vi "gyro-sweeper-V3.vi"() -> ()   [LabVIEW 2018]
uses:
  filename-pattern.ctl
  show-win- control.ctl
  cursor winow.ctl
  cursor window action.ctl
  server talkto message type.ctl
  server talkback message type.ctl
  server talk-to-back pair.ctl
  pll internal user event action.ctl
  publisher action.ctl
  file -- read-write control.ctl
  KM_file -- read-write control.ctl
  filename-action.ctl
  <vilib>/Analysis/baseanly.llb/A x B.vi
  <vilib>/Analysis/baseanly.llb/Complex A x B.vi
  Q -- check range -- i -- real.vi
  line -- complex.vi
  Q -- check range -- i -- integer.vi
  Q - not nan -- real.vi
  Q - not nan -- integer.vi
  <vilib>/Analysis/Matrix/Numeric/Conversions/Array To Matrix.vi
  <vilib>/Analysis/Matrix/Numeric/Conversions/Array To Matrix - RA2.vi
  <vilib>/Analysis/baseanly.llb/Inverse Matrix.vi
  <vilib>/Analysis/baseanly.llb/Real Inverse Matrix.vi
panel:
  in  "(*) sourcer":bool
  in  "exit!":bool
  in  "(*) fitter":bool
  in  "(*) sweeper":bool=TRUE
  in  "sweeper panel":T1(tab)
  in  "sweep is ON":bool
  in  "win":T2={"cen (Hz)"=32754.180483243686, "win (Hz)"=308.86311527720136, "left (Hz)"=32599.748925605087, "right (Hz)"=32908.61204088229}
  out "Plot: circle sweep window":cluster{"Freq out (Hz)":dbl[], dbl[]}[](graph)
  in  "sweep! :r":bool
  in  "subtract bgnd!":bool
  in  "fit!":bool=TRUE
  in  "cursor window":T3={"left"=32599.748925605087, "right "=32908.61204088229, "center"=32754.180483243686, "window"=308.86311527720136, "cursors"=[0, 1, 2], "relative"=0, "absolute"=0, "fixed vertical offset"=0.0, "vertical offset"=0.0, "skew"=0.0, "default window frac"=0.1, "kind"=enum."symmetric", "skew.left"=0.5, "skew.right"=0.5, "Plot ref"=refnum, "wing order"=enum."forw"}
  out "async sweeper":refnum<vi>
  out "async fitter":refnum<vi>
  out "async sourcer":refnum<vi>
  in  "view/hide sweeper 2":bool=TRUE
  in  "view/hide fitter 2":bool
  in  "view/hide sourcer 2":bool
  in  "save data":enum32{"save/read"}(tab)
  in  "freqsweep name template":T4={"prefix"="RuCl3-rod", "group"="f"}
  in  "Save folder":path=path "/Users/Shared/Data"
  in  "freq sweep file name":string="f020_RuCl3-rod_042518.dat"
  in  "read from disk :l":bool
  in  "read file":path=path "/Users/arkady/Desktop/local_data/TaAs-quirk-Jan2018-losalamos/9w/f006_rucl3_012518.dat"
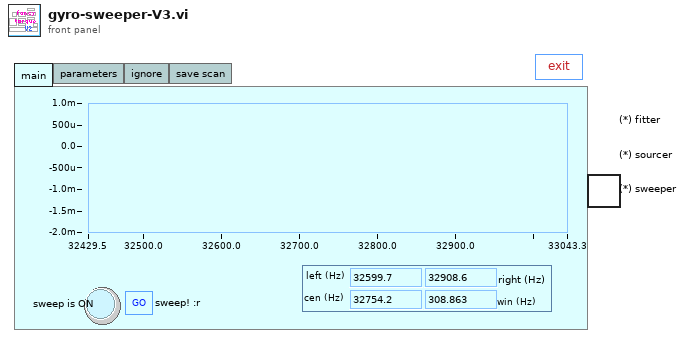
[diagram p1: front panel]
types:
  T1 = enum32{"main", "parameters", "ignore", "save scan"}
  T2 = typedef "show-win- control.ctl" = cluster{"cen (Hz)":dbl, "win (Hz)":dbl, "left (Hz)":dbl, "right (Hz)":dbl}
  T3 = typedef "cursor winow.ctl" = cluster{"left":dbl, "right ":dbl, "center":dbl, "window":dbl, "cursors":i32[], "relative":i32, "absolute":i32, "fixed vertical offset":dbl, "vertical offset":dbl, "skew":dbl, "default window frac":dbl, "kind":enum16{"symmetric", "skewed", "fancy"}, "skew.left":dbl, "skew.right":dbl, "Plot ref":refnum<vi>, "wing order":enum16{"forw", "back"}}
  T4 = typedef "filename-pattern.ctl" = cluster{"prefix":string, "group":string}
  T5 = typedef "server talk-to-back pair.ctl" = cluster{"talkback event":refnum<user-event>, "talkto event":refnum<user-event>}
  T6 = typedef "server talkback message type.ctl" = cluster{"message":enum16{"new"}}
  T7 = typedef "server talkto message type.ctl" = cluster{"message":enum16{"stop", "start", "update pars", "update request", "new", "launch", "exit", "get", "reset", "pause", "unpause"}}
  T8 = typedef "pll internal user event action.ctl" = enum16{"gear pll async", "start pll async", "stop pll async", "toggle pll async", "gear sweeper", "start sweeper", "stop sweeper", "toggle sweeper", "accept frequency", "reset lorentzian", "accept lorentzian", "update cursors", "pause pll", "unpause pll", "void"}
  T9 = typedef "cursor window action.ctl" = enum16{"balance", "h. offset change", "cursor moves", "change center", "change window", "init", "check", "reset", "set y to middle", "idle", "-write all Y", "-write left.X", "-write center.X", "-write right.X", "-write all X", "-change center", "-change window", "-change skew", "-read cursor 2", "-read cursor 1", "-read cursor 0", "-read all cursors", "-reset", "-read plot scale", "-set y to middle", "-Q: center.Y is visible", "-Q: window is visible", "-parse center.Y", "-right left from center", "-left move", "-right move", "-set center.Y", "-empty", "-set cursors to default", "-check", "-write center.Y", "-copy cursor 1", "-copy cursor 0", "-copy cursor 2", "move right", "move left", "shrink", "broaden", "skew up", "skew down", "-write plot scale", "zoom X", "change cen&win", "zoom to all data", "color--red", "color--green", "color--yellow", "read", "zoom out", "zoom in", "slide right", "slide left", "set range aspect ratio to 1"}
  T10 = typedef "eventvkey.ctl" = enum16{"ASCII", "Enter", "Return", "Shift", "Ctrl", "Alt", "Cmd", "Opt", "Caps", "NumLock", "Clear", "Break", "Up", "Down", "Left", "Right", "Insert", "Delete", "Home", "End", "PageUp", "PageDown", "Escape", "Help", "Pause", "ScrollLock", "F1", "F2", "F3", "F4", "F5", "F6", "F7", "F8", "F9", "F10", "F11", "F12", "F13", "F14", "F15", "F16", "F17", "F18", "F19", "F20", "F21", "F22", "F23", "F24", "Play", "VolumeUp", "VolumeDown", "Mute", "Two Byte Char"}
  T11 = typedef "publisher action.ctl" = enum16{"set", "get", "init", "check"}
  T12 = typedef "file -- read-write control.ctl" = enum16{"read", "write all", "append one line"}
  T13 = typedef "filename-action.ctl" = enum16{"rewrite", "parse", "force pattern", "uniquenum"}
  T14 = typedef "KM_file -- read-write control.ctl" = enum16{"read", "write all", "append one line"}
  T15 = enum32{"Invalid", "Standard", "Closed", "Hidden", "Minimized", "Maximized"}
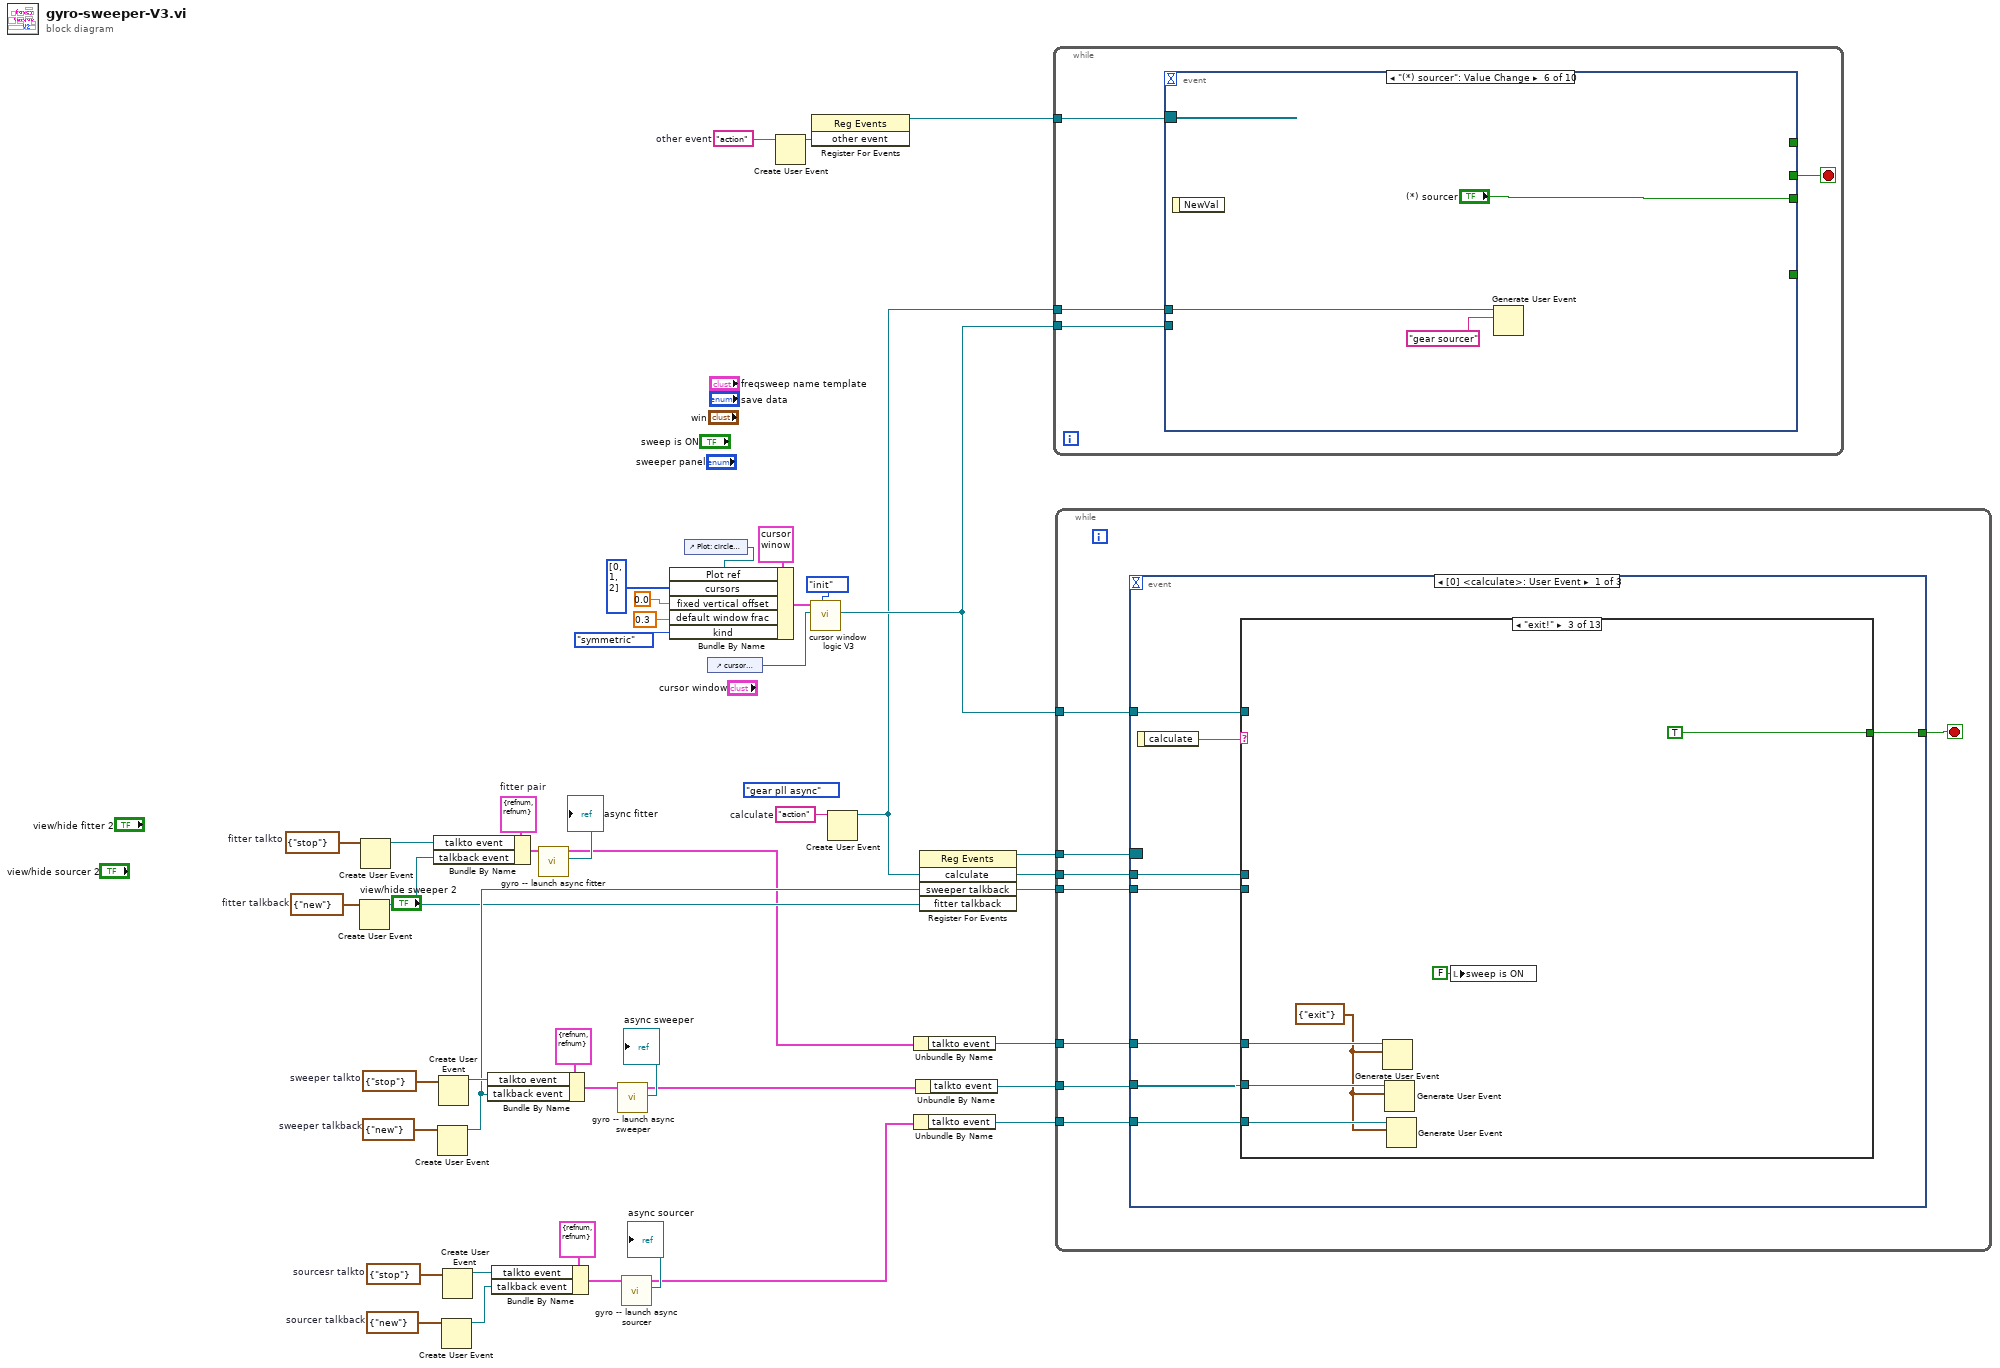
[diagram p0: block diagram]
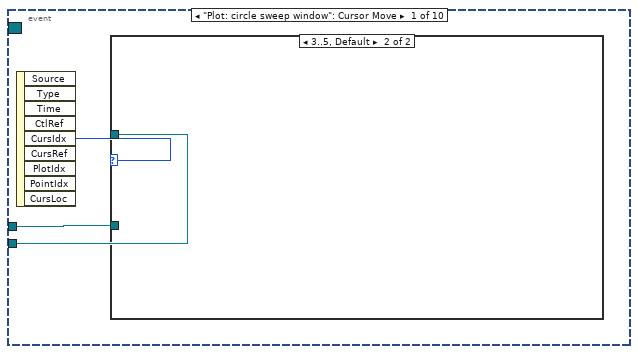
[diagram p2: hidden frame]
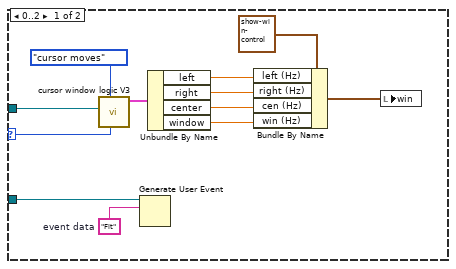
[diagram p3: hidden frame]
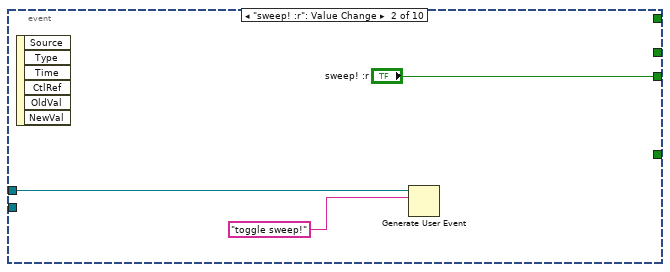
[diagram p4: hidden frame]
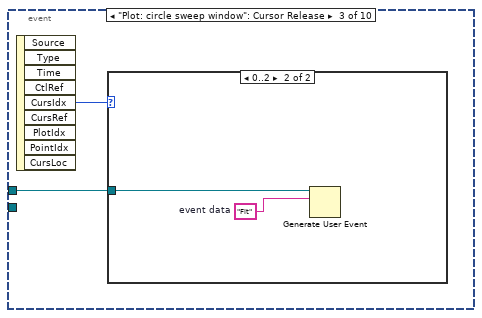
[diagram p5: hidden frame]
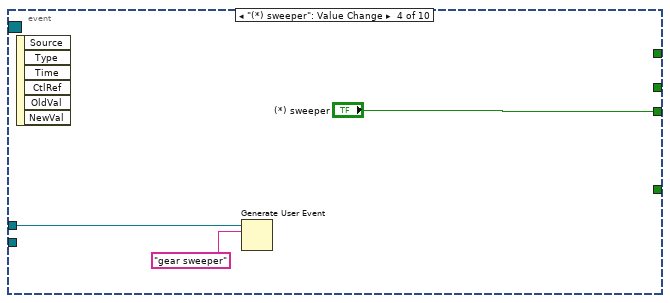
[diagram p7: hidden frame]
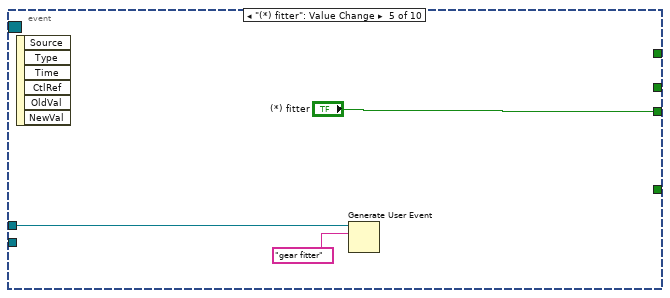
[diagram p8: hidden frame]
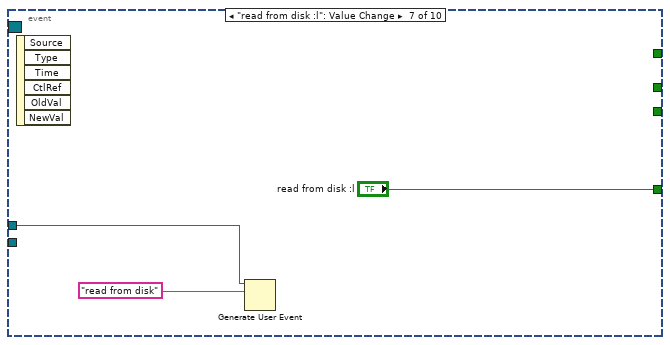
[diagram p9: hidden frame]
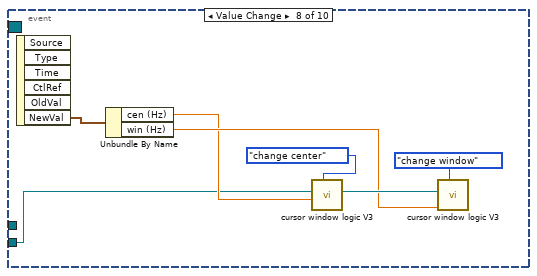
[diagram p10: hidden frame]
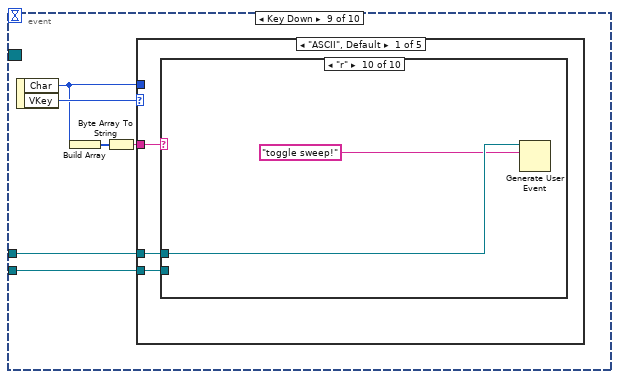
[diagram p11: hidden frame]
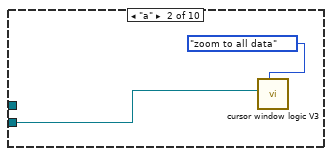
[diagram p13: hidden frame]
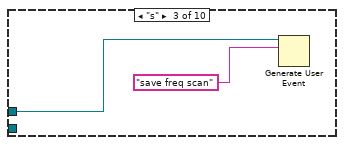
[diagram p14: hidden frame]
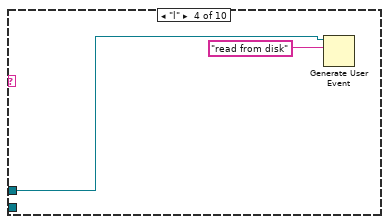
[diagram p15: hidden frame]
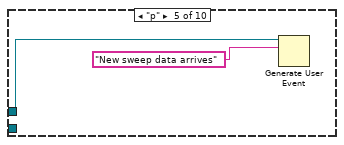
[diagram p16: hidden frame]
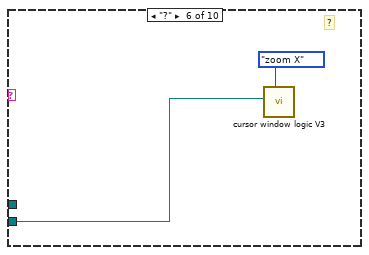
[diagram p17: hidden frame]
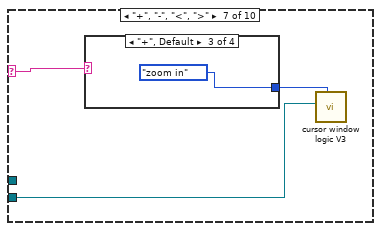
[diagram p18: hidden frame]
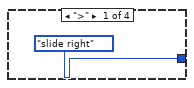
[diagram p19: hidden frame]
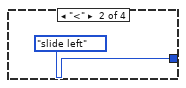
[diagram p20: hidden frame]
diagram:
  w5 = T6 {"message"=enum."new"}  # sourcer talkback
  w6 = T7 {"message"=enum."stop"}  # sourcesr talkto
  w17 = T6 {"message"=enum."new"}  # sweeper talkback
  w18 = T7 {"message"=enum."stop"}  # sweeper talkto
  w26 = T5 {"talkback event"=refnum, "talkto event"=refnum}  # fitter pair
  w15 = T6 {"message"=enum."new"}  # fitter talkback
  w16 = T7 {"message"=enum."stop"}  # fitter talkto
  (unwired) pll_internal_user_event_action."gear pll async" ("pll event action")
  w40 = "action"  # other event
  w42 = "action"  # calculate
  n1 = Create User Event(user event datatype=w15) -> (user event=w12:refnum<user-event>)  [unwired: 1 in, 1 out]
  n2 = Create User Event(user event datatype=w16) -> (user event=w25:refnum<user-event>)  [unwired: 1 in, 1 out]
  n3 = Bundle By Name(cluster=w26, "talkto event"=w25, "talkback event"=w12) -> (w19:T5)
  n4 = Create User Event(user event datatype=w17) -> (user event=w13:refnum<user-event>)  [unwired: 1 in, 1 out]
  n5 = Create User Event(user event datatype=w18) -> (user event=w23:refnum<user-event>)  [unwired: 1 in, 1 out]
  n6 = Create User Event(user event datatype=w5) -> (user event=w3:refnum<user-event>)  [unwired: 1 in, 1 out]
  n7 = Create User Event(user event datatype=w6) -> (user event=w8:refnum<user-event>)  [unwired: 1 in, 1 out]
  n8 = Bundle By Name(cluster=T5 {"talkback event"=refnum, "talkto event"=refnum} ("sweeper pair"), "talkto event"=w23, "talkback event"=w13) -> (w14:T5)
  n9 = Bundle By Name(cluster=T5 {"talkback event"=refnum, "talkto event"=refnum} ("sweeper pair"), "talkto event"=w8, "talkback event"=w3) -> (w4:T5)
  n10 = call "gyro -- launch async fitter.vi"("fitter pair"=w19) -> ("reference out"=→"async fitter":refnum<vi>, "fitter pair OUT"=w10:T5)  [unwired: 9 in]
  n11 = call "gyro -- launch async sweeper.vi"("sweeper event pair"=w14) -> ("reference out"=→"async sweeper":refnum<vi>, "sweeper event pair OUT"=w11:T5)  [unwired: 9 in]
  n12 = call "gyro -- launch async sourcer.vi"("sourcer pair"=w4) -> ("reference out"=→"async sourcer":refnum<vi>, "fitter pair OUT"=w2:T5)  [unwired: 9 in]
  n13 = control-ref of="Plot: circle sweep window"() -> (w29:refnum<vi>)
  n14 = Bundle By Name(cluster=T3 {"left"=0.0, "right "=0.0, "center"=0.0, "window"=0.0, "cursors"=[], "relative"=0, "absolute"=0, "fixed vertical offset"=0.0, "vertical offset"=0.0, "skew"=0.0, "default window frac"=0.0, "kind"=enum."symmetric", "skew.left"=0.0, "skew.right"=0.0, "Plot ref"=refnum, "wing order"=enum."forw"} ("cursor bracket: All, data window"), "Plot ref"=w29, "cursors"=i32[] [0, 1, 2], "fixed vertical offset"=0.0, "default window frac"=0.3 ("fixed vertical offset"), "kind"=enum16{"symmetric", "skewed", "fancy"}."symmetric") -> (w34:T3)
  n15 = control-ref of="cursor window"() -> (w27:refnum<vi>)
  n16 = Create User Event(user event datatype=w40) -> (user event=w39:refnum<user-event>)  [unwired: 1 in, 1 out]
  n17 = call "cursor window logic V3.vi"("cursor window action"=cursor_window_action."init", "cursor window in"=w27, "cursor window init"=w34) -> ("cursor window out"=w32:refnum<vi>)  [unwired: 7 in, 1 out]
  n18 = register-events(w39) -> (reference out=w41:refnum<event-registration>)  [unwired: 2 in, 1 out]
  n19 = Create User Event(user event datatype=w42) -> (user event=w30:refnum<user-event>)  [unwired: 1 in, 1 out]
  n20 = Unbundle By Name(w10) -> ("talkto event"=w21:refnum<user-event>)
  n21 = Unbundle By Name(w2) -> ("talkto event"=w1:refnum<user-event>)
  n22 = Unbundle By Name(w11) -> ("talkto event"=w22:refnum<user-event>)
  n23 = register-events(w30, w13, w12) -> (reference out=w43:refnum<event-registration>)  [unwired: 2 in, 1 out]
  n24 = while {
    tunnel: w41 -> [w47]
    tunnel: w30 -> [w46]
    tunnel: w32 -> [w45]
    stop <- w44 stop-if-true
    n25 = event shown="[5] \"(*) sourcer\": Value Change" {
      selector: w47 -> [_ _ _ _ _ _ _ _ _ _]
      dyn-events: _ -> [_ _ _ _ _ _ _ _ _ _]
      timeout: _ -> [_ _ _ _ _ _ _ _ _ _]
      tunnel: w46 -> [w48 w64 w67 w71 w73 w76 w81 _ w93 w138]
      tunnel: w45 -> [w50 _ _ _ _ _ _ w82 w89 _]
      tunnel: [_ "sweep! :r" _ "(*) sweeper" "(*) fitter" "(*) sourcer" _ _ _ _] -> _
      tunnel: [_ _ _ _ _ _ "read from disk :l" _ _ _] -> _
      tunnel: [_ _ _ _ _ _ _ _ _ "exit!"] -> _
      tunnel: [_ _ _ _ _ _ _ _ _ TRUE] -> w44
      event "Plot: circle sweep window": Cursor Move {
        n26 = event-data() -> ("CursIdx"=w49:i32)  [unwired: 1 in, 8 out]
        n27 = case shown="3..5, Default" w49 {
          selector: w49 -> [w60 _]
          tunnel: w50 -> [w62 _]
          tunnel: w48 -> [w58 _]
          frame 0..2 {
            w57 = "Fit"  # event data
            n28 = call "cursor window logic V3.vi"("CursIdx"=w60, "cursor window action"=cursor_window_action."cursor moves", "cursor window in"=w62) -> ("cursor window out"=w59:T3)  [unwired: 7 in, 1 out]
            n29 = Generate User Event(user event=w58, event data cluster=w57) -> ()  [unwired: 2 in, 2 out]
            n30 = Unbundle By Name(w59) -> ("left"=w54:dbl, "right"=w53:dbl, "center"=w52:dbl, "window"=w51:dbl)
            n31 = Bundle By Name(cluster=T2 {"cen (Hz)"=-0.35260838541595674, "win (Hz)"=17.234446484426172, "left (Hz)"=-8.969831627629043, "right (Hz)"=8.26461485679713} ("win"), "left (Hz)"=w54, "right (Hz)"=w53, "cen (Hz)"=w52, "win (Hz)"=w51) -> (w55:T2)
            n32 = local write "win"(w55) -> ()
          }
          frame 3..5, Default {
          }
        }
      }
      event "sweep! :r": Value Change {
        n33 = event-data() -> ()  [unwired: 1 in, 6 out]
        n34 = Generate User Event(user event=w64, event data cluster="toggle sweep!" ("event data")) -> ()  [unwired: 2 in, 2 out]
      }
      event "Plot: circle sweep window": Cursor Release {
        n35 = event-data() -> ("CursIdx"=w66:i32)  [unwired: 1 in, 8 out]
        n36 = case shown="0..2" w66 {
          tunnel: w67 -> [_ w68]
          frame 3, Default {
          }
          frame 0..2 {
            w69 = "Fit"  # event data
            n37 = Generate User Event(user event=w68, event data cluster=w69) -> ()  [unwired: 2 in, 2 out]
          }
        }
      }
      event "(*) sweeper": Value Change {
        n38 = event-data() -> ()  [unwired: 1 in, 6 out]
        n39 = Generate User Event(user event=w71, event data cluster="gear sweeper" ("event data")) -> ()  [unwired: 2 in, 2 out]
      }
      event "(*) fitter": Value Change {
        n40 = event-data() -> ()  [unwired: 1 in, 6 out]
        n41 = Generate User Event(user event=w73, event data cluster="gear fitter" ("event data")) -> ()  [unwired: 2 in, 2 out]
      }
      event "(*) sourcer": Value Change {
        n42 = event-data() -> ()  [unwired: 1 in, 1 out]
        n43 = Generate User Event(user event=w76, event data cluster="gear sourcer" ("event data")) -> ()  [unwired: 2 in, 2 out]
      }
      event "read from disk :l": Value Change {
        n44 = event-data() -> ()  [unwired: 1 in, 6 out]
        n45 = Generate User Event(user event=w81, event data cluster="read from disk" ("event data")) -> ()  [unwired: 2 in, 2 out]
      }
      event Value Change {
        n46 = event-data() -> ("NewVal"=w85:T2)  [unwired: 1 in, 5 out]
        n47 = Unbundle By Name(w85) -> ("cen (Hz)"=w83:dbl, "win (Hz)"=w84:dbl)
        n48 = call "cursor window logic V3.vi"("cursor window action"=cursor_window_action."change center", "center"=w83, "cursor window in"=w82) -> ("cursor window out"=w86:refnum<vi>)  [unwired: 7 in, 1 out]
        n49 = call "cursor window logic V3.vi"("cursor window action"=cursor_window_action."change window", "window"=w84, "cursor window in"=w86) -> ()  [unwired: 7 in, 2 out]
      }
      event Key Down {
        n50 = event-data() -> ("Char"=w91:i16, "VKey"=w94:T10)  [unwired: 1 in]
        n51 = Build Array(w91) -> (w92:i16[])
        n52 = Byte Array To String(unsigned byte array=w92) -> (string=w90:string)
        n53 = case shown="\"ASCII\", Default" w94 {
          selector: w94 -> [_ _ _ _ w132]
          tunnel: w91 -> [_ _ _ _ _]
          tunnel: w93 -> [w97 _ _ _ w131]
          tunnel: w90 -> [w96 _ _ _ _]
          tunnel: w89 -> [w95 _ _ _ w128]
          frame "ASCII", Default {
            n54 = case shown="\"r\"" w96 {
              selector: w96 -> [_ _ _ _ _ _ w109 _ _ _]
              tunnel: w97 -> [_ _ w100 w102 w104 _ _ _ _ w118]
              tunnel: w95 -> [_ w98 _ _ _ w106 w110 w115 _ _]
              frame "0", Default {
              }
              frame "a" {
                n55 = call "cursor window logic V3.vi"("cursor window action"=cursor_window_action."zoom to all data", "cursor window in"=w98) -> ()  [unwired: 8 in, 2 out]
              }
              frame "s" {
                n56 = Generate User Event(user event=w100, event data cluster="save freq scan" ("event data")) -> ()  [unwired: 2 in, 2 out]
              }
              frame "l" {
                n57 = Generate User Event(user event=w102, event data cluster="read from disk" ("event data")) -> ()  [unwired: 2 in, 2 out]
              }
              frame "p" {
                n58 = Generate User Event(user event=w104, event data cluster="New sweep data arrives" ("event data")) -> ()  [unwired: 2 in, 2 out]
              }
              frame "?" {
                # "?"
                n59 = call "cursor window logic V3.vi"("cursor window action"=cursor_window_action."zoom X", "cursor window in"=w106) -> ()  [unwired: 8 in, 2 out]
              }
              frame "+", "-", "<", ">" {
                n60 = case shown="\"+\", Default" w109 {
                  tunnel: [cursor_window_action."slide right" ("cursor window action") cursor_window_action."slide left" ("cursor window action") cursor_window_action."zoom in" ("cursor window action") cursor_window_action."zoom out" ("cursor window action")] -> w108
                  frame ">" {
                  }
                  frame "<" {
                  }
                  frame "+", Default {
                  }
                  frame "-" {
                  }
                }
                n61 = call "cursor window logic V3.vi"("cursor window action"=w108, "cursor window in"=w110) -> ()  [unwired: 8 in, 2 out]
              }
              frame "c" {
                n62 = call "cursor window logic V3.vi"("cursor window action"=cursor_window_action."check", "cursor window in"=w115) -> ()  [unwired: 8 in, 2 out]
              }
              frame "t" {
              }
              frame "r" {
                n63 = Generate User Event(user event=w118, event data cluster="toggle sweep!" ("event data")) -> ()  [unwired: 2 in, 2 out]
              }
            }
          }
          frame "Escape" {
          }
          frame "PageUp" {
          }
          frame "PageDown" {
          }
          frame "Up".."Right" {
            w119 = "update win"  # event data
            w121 = "Fit"  # event data
            n64 = case shown="\"Left\"" w132 {
              tunnel: [cursor_window_action."move right" ("cursor window action") cursor_window_action."move left" ("cursor window action") cursor_window_action."broaden" ("cursor window action") cursor_window_action."shrink" ("cursor window action")] -> w130
              frame "Right", Default {
              }
              frame "Left" {
              }
              frame "Up" {
              }
              frame "Down" {
              }
            }
            n65 = call "cursor window logic V3.vi"("cursor window action"=w130, "cursor window in"=w128) -> ("cursor window out"=w129:T3)  [unwired: 8 in, 1 out]
            n66 = Unbundle By Name(w129) -> ("left"=w125:dbl, "right"=w124:dbl, "center"=w123:dbl, "window"=w122:dbl)
            n67 = Generate User Event(user event=w131, event data cluster=w121) -> (user event out=w120:refnum<user-event>)  [unwired: 2 in, 1 out]
            n68 = Bundle By Name(cluster=T2 {"cen (Hz)"=-0.35260838541595674, "win (Hz)"=17.234446484426172, "left (Hz)"=-8.969831627629043, "right (Hz)"=8.26461485679713} ("win"), "left (Hz)"=w125, "right (Hz)"=w124, "cen (Hz)"=w123, "win (Hz)"=w122) -> (w127:T2)
            n69 = Generate User Event(user event=w120, event data cluster=w119) -> ()  [unwired: 2 in, 2 out]
            n70 = local write "win"(w127) -> ()
          }
        }
      }
      event "exit!": Value Change {
        n71 = event-data() -> ()  [unwired: 1 in, 6 out]
        n72 = Generate User Event(user event=w138, event data cluster="exit!" ("event data")) -> ()  [unwired: 2 in, 2 out]
      }
    }
  }
  n73 = while {
    tunnel: w43 -> [w148]
    tunnel: w30 -> [w147]
    tunnel: w32 -> [w146]
    tunnel: w22 -> [w145]
    tunnel: w13 -> [w144]
    tunnel: w21 -> [w143]
    tunnel: w1 -> [w141]
    stop <- w142 stop-if-true
    n74 = event shown="[0] <calculate>: User Event" {
      selector: w148 -> [_ _ _]
      dyn-events: _ -> [_ _ _]
      timeout: _ -> [_ _ _]
      tunnel: w147 -> [w155 w270 _]
      tunnel: w146 -> [w154 _ _]
      tunnel: w145 -> [w153 _ _]
      tunnel: w144 -> [w152 _ _]
      tunnel: w143 -> [w151 _ _]
      tunnel: [w150 _ _] -> w142
      tunnel: w141 -> [w149 _ _]
      event User Event {
        n75 = event-data() -> ("calculate"=w156:string)  [unwired: 1 in]
        n76 = case shown="\"exit!\"" w156 {
          tunnel: w155 -> [w165 w188 _ w197 _ _ _ _ _ _ _ _ _]
          tunnel: w154 -> [_ _ _ _ _ w229 _ _ _ _ _ _ _]
          tunnel: w153 -> [_ _ w195 _ _ _ w242 w247 w251 _ _ _ _]
          tunnel: w152 -> [_ _ _ _ _ _ _ _ _ _ _ _ _]
          tunnel: w151 -> [_ _ w194 _ _ w227 _ _ _ _ _ _ _]
          tunnel: [_ _ TRUE _ _ _ _ _ _ _ _ _ _] -> w150
          tunnel: w149 -> [_ _ w192 _ _ _ _ _ _ _ _ _ _]
          frame "New sweep data arrives" {
            n77 = call "MFLI -- publish -- freq scan.vi"("publisher action"=publisher_action."get") -> ("Voltage out (V)"=w162:cdb[], "Freq out (Hz)"=w164:dbl[])  [unwired: 9 in]
            n78 = Generate User Event(user event=w165, event data cluster="Fit" ("event data")) -> ()  [unwired: 2 in, 2 out]
            n79 = case shown="False" "subtract bgnd!" {
              tunnel: w164 -> [w177 w185]
              tunnel: [w171 w185] -> w163
              tunnel: w162 -> [w173 w184]
              tunnel: [w178 w184] -> w161
              frame True {
                w170 = 10 ("length")
                n80 = Delete From Array(array=w177, length=w170, index=0) -> (array with subset deleted=w176:dbl[])  [unwired: 1 out]
                n81 = Delete From Array(array=w173, length=w170, index=0) -> (array with subset deleted=w172:cdb[])  [unwired: 1 out]
                n82 = call "linear interp iiii- complex - z-omega.vi"("z"=w172, "omega"=w176) -> ("z out"=w179:cdb[], "omega out"=w171:dbl[], "intercept"=w181:cdb, "slope"=w182:cdb)  [unwired: 5 in, 5 out]
                n83 = Multiply(x=w171, y=w182) -> (x*y=w183:cdb[])
                n84 = Add(x=w183, y=w181) -> (x+y=w180:cdb[])
                n85 = Subtract(x=w179, y=w180) -> (x-y=w178:cdb[])
              }
              frame False {
              }
            }
            n86 = Complex To Re/Im(x + iy=w161) -> (x=w168:dbl[], y=w167:dbl[])
            n87 = Bundle("Freq out (Hz)"=w163, w168) -> (w169:cluster{"Freq out (Hz)":dbl[], dbl[]})  [unwired: 1 in]
            n88 = Bundle("Freq out (Hz)"=w163, w167) -> (w166:cluster{"Freq out (Hz)":dbl[], dbl[]})  [unwired: 1 in]
            n89 = Build Array(w169, w166) -> (→"Plot: circle sweep window":cluster{"Freq out (Hz)":dbl[], dbl[]}[])
          }
          frame "toggle sweep!" {
            n90 = local read "sweep is ON"() -> (w187:bool)
            n91 = case shown="False" w187 {
              tunnel: ["start sweep!" ("event data") "stop sweep!" ("event data")] -> w186
              frame False {
              }
              frame True {
              }
            }
            n92 = Generate User Event(user event=w188, event data cluster=w186) -> ()  [unwired: 2 in, 2 out]
          }
          frame "exit!" {
            w191 = T7 {"message"=enum."exit"} ("event data")
            n93 = Generate User Event(user event=w194, event data cluster=w191) -> ()  [unwired: 2 in, 2 out]
            n94 = Generate User Event(user event=w195, event data cluster=w191) -> ()  [unwired: 2 in, 2 out]
            n95 = Generate User Event(user event=w192, event data cluster=w191) -> ()  [unwired: 2 in, 2 out]
            n96 = local write "sweep is ON"(FALSE ("sweep ON")) -> ()
          }
          frame "read from disk" {
            n97 = call "file - read-write - list of lines.vi"("read/write control"=file_--_read-write_control."read", "file path"="read file") -> ("list of lines OUT"=w201:string[])  [unwired: 8 in, 1 out]
            n98 = for {
              tunnel: w201 -> [w211] mode=indexing
              tunnel: [w206] -> w202 mode=indexing
              tunnel: [w205] -> w203 mode=indexing
              w207 = 0.0
              n99 = Scan From String(format string="%f%f%f", input string=w211, default 1=w207, default 2=w207, default 3=w207) -> (output 1=w205:dbl, output 2=w209:dbl, output 3=w208:dbl)  [unwired: 2 in, 3 out]
              n100 = Re/Im To Complex(1:w208, 2:w209) -> (0:w206:cdb)
            }
            n101 = flat-sequence {
              tunnel: w197 -> [w215]
              tunnel: [w215] -> w204
              tunnel: w202 -> [w213]
              tunnel: w203 -> [w212]
              tunnel: w204 -> [w217]
              tunnel: "New sweep data arrives" ("event data") -> [w216]
              frame #0 {
                n102 = call "MFLI -- publish -- freq scan.vi"("publisher action"=publisher_action."set", "Voltage IN (V)"=w213, "Freq IN (Hz)"=w212) -> ()  [unwired: 7 in, 2 out]
              }
              frame #1 {
                n103 = Generate User Event(user event=w217, event data cluster=w216) -> ()  [unwired: 2 in, 2 out]
              }
            }
          }
          frame "save freq scan" {
            n104 = local read "freqsweep name template"() -> (w223:T4)
            n105 = call "MFLI -- publish -- freq scan.vi"("publisher action"=publisher_action."get") -> ("Voltage out (V)"=w219:cdb[], "Freq out (Hz)"=w220:dbl[])  [unwired: 9 in]
            n106 = call "filename-manage.vi"("filename pattern"=w223, "filename-action"=filename-action."uniquenum", "folder"="Save folder", "file name"="freq sweep file name") -> ("filename OUT"=w222:string)  [unwired: 7 in]
            n107 = call "KM_appendline -- freq sweep.vi"("freq"=w220, "Vout(V)"=w219, "Save frequency scan"="Save folder", "read/write control"=KM_file_--_read-write_control."append one line", "name or relative path"=w222) -> ()  [unwired: 15 in]
            n108 = local write "freq sweep file name"(w222) -> ()
          }
          frame "Fit" {
            n109 = case shown="True" "fit!" {
              tunnel: w229 -> [_ w231]
              tunnel: w227 -> [_ w230]
              frame False {
              }
              frame True {
                n110 = flat-sequence {
                  tunnel: w231 -> [w234]
                  tunnel: w230 -> [w236]
                  frame #0 {
                    n111 = call "cursor window logic V3.vi"("cursor window action"=cursor_window_action."read", "cursor window in"=w234) -> ("cursor window out"=w233:T3)  [unwired: 8 in, 1 out]
                    n112 = call "publish -- fitter window.vi"("publisher action"=publisher_action."set", "win IN"=w233) -> ()  [unwired: 9 in, 1 out]
                  }
                  frame #1 {
                    n113 = Generate User Event(user event=w236, event data cluster=T7 {"message"=enum."new"} ("event data")) -> ()  [unwired: 2 in, 2 out]
                  }
                }
              }
            }
          }
          frame "start sweep!" {
            n114 = local read "win"() -> (w239:T2)
            n115 = call "publish -- sweeper window.vi"("publisher action"=publisher_action."set", "win IN"=w239) -> ()  [unwired: 9 in, 1 out]
            n116 = local write "sweep is ON"(TRUE ("sweep ON")) -> ()
            n117 = Generate User Event(user event=w242, event data cluster=T7 {"message"=enum."update request"} ("event data")) -> (user event out=w241:refnum<user-event>)  [unwired: 2 in, 1 out]
            n118 = Generate User Event(user event=w241, event data cluster=T7 {"message"=enum."start"} ("event data")) -> ()  [unwired: 2 in, 2 out]
          }
          frame "stop sweep!" {
            n119 = Generate User Event(user event=w247, event data cluster=T7 {"message"=enum."stop"} ("event data")) -> ()  [unwired: 2 in, 2 out]
            n120 = local write "sweep is ON"(FALSE ("sweep ON")) -> ()
          }
          frame "update win" {
            n121 = local read "win"() -> (w248:T2)
            n122 = call "publish -- sweeper window.vi"("publisher action"=publisher_action."set", "win IN"=w248) -> ()  [unwired: 9 in, 1 out]
            n123 = Generate User Event(user event=w251, event data cluster=T7 {"message"=enum."update request"} ("event data")) -> ()  [unwired: 2 in, 2 out]
          }
          frame "gear sweeper" {
            n124 = local read "async sweeper"() -> (w253:refnum<vi>)
            n125 = property class="VI Interface Type 0"(reference=w253) -> ("FP.State"=w252:T15)  [unwired: 1 in, 2 out]
            n126 = case shown="\"Closed\"" w252 {
              tunnel: w253 -> [w256 w257]
              frame "Closed" {
                n127 = invoke class="VI (strict)" method="FP.Open"(reference=w256, "Activate"=TRUE ("Activate?"), "State"=T15."Standard" ("Front Panel Window:State")) -> ()  [unwired: 2 in, 5 out]
              }
              frame "Standard", Default {
                n128 = invoke class="VI (strict)" method="FP.Close"(reference=w257) -> ()  [unwired: 2 in, 3 out]
              }
            }
          }
          frame "gear sourcer" {
            n129 = local read "async sourcer"() -> (w259:refnum<vi>)
            n130 = property class="VI Interface Type 0"(reference=w259) -> ("FP.State"=w258:T15)  [unwired: 1 in, 2 out]
            n131 = case shown="\"Closed\"" w258 {
              tunnel: w259 -> [w262 w263]
              frame "Closed" {
                n132 = invoke class="VI (strict)" method="FP.Open"(reference=w262, "Activate"=TRUE ("Activate?"), "State"=T15."Standard" ("Front Panel Window:State")) -> ()  [unwired: 2 in, 5 out]
              }
              frame "Standard", Default {
                n133 = invoke class="VI (strict)" method="FP.Close"(reference=w263) -> ()  [unwired: 2 in, 3 out]
              }
            }
          }
          frame "gear fitter" {
            n134 = local read "async fitter"() -> (w265:refnum<vi>)
            n135 = property class="VI Interface Type 0"(reference=w265) -> ("FP.State"=w264:T15)  [unwired: 1 in, 2 out]
            n136 = case shown="\"Closed\"" w264 {
              tunnel: w265 -> [w268 w269]
              frame "Closed" {
                n137 = invoke class="VI (strict)" method="FP.Open"(reference=w268, "Activate"=TRUE ("Activate?"), "State"=T15."Standard" ("Front Panel Window:State")) -> ()  [unwired: 2 in, 5 out]
              }
              frame "Standard", Default {
                n138 = invoke class="VI (strict)" method="FP.Close"(reference=w269) -> ()  [unwired: 2 in, 3 out]
              }
            }
          }
          frame "Void", Default {
          }
        }
      }
      event User Event {
        n139 = event-data() -> ("message"=w271:enum16{"new"})  [unwired: 1 in, 4 out]
        n140 = case shown="\"new\", Default" w271 {
          tunnel: w270 -> [w272]
          frame "new", Default {
            n141 = Generate User Event(user event=w272, event data cluster="New sweep data arrives" ("event data")) -> ()  [unwired: 2 in, 2 out]
          }
        }
      }
      event User Event {
        n142 = event-data() -> ()  [unwired: 1 in, 1 out]
      }
    }
  }
